vi "test_proceed.vi"() -> ()   [LabVIEW 2013]
uses:
  Classes/Flags/flag.lvclass
  global variables.vi
panel:
  in  "notifier name":string="test"
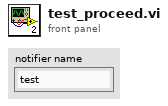
[diagram p1: front panel]
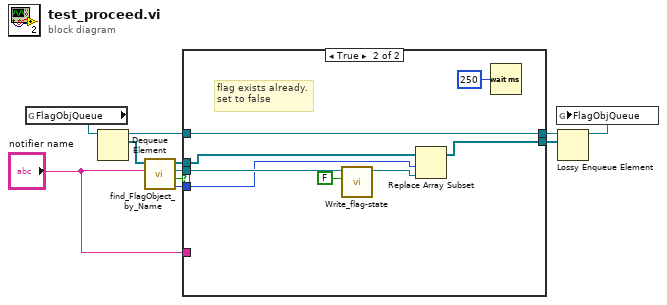
[diagram p0: block diagram]
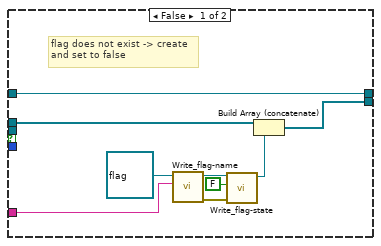
[diagram p2: hidden frame]
diagram:
  n1 = global read "global variables.vi" "FlagObjQueue"() -> (w11:refnum<queue>)
  n2 = Dequeue Element(queue=w11) -> (queue out=w9:refnum<queue>, element=w4:refnum<class "flag.lvclass">[])  [unwired: 2 in, 2 out]
  n3 = call "find_FlagObject_by_Name.vi"("Flag Name"="notifier name", "FlagObj Array"=w4) -> ("index of Object in Array"=w2:i32, "found?"=w10:bool, "found FlagObj out"=w7:refnum<class "flag.lvclass">, "FlagObj Array out"=w8:refnum<class "flag.lvclass">[])  [unwired: 6 in]
  n4 = case shown="True" w10 {
    tunnel: w9 -> [w13 w27]
    tunnel: w8 -> [w19 w24]
    tunnel: "notifier name" -> [w20 _]
    tunnel: w7 -> [_ w26]
    tunnel: [w13 w27] -> w6
    tunnel: [w12 w21] -> w5
    tunnel: w2 -> [_ w22]
    frame False {
      # "flag does not exist -> create\nand set to false"
      n5 = call-dynamic "Write_flag-name.vi"("flag name"=w20, "flag in"=refnum<class "flag.lvclass"> refnum ("flag.lvclass")) -> ("error out"=w16:errorcluster, "flag out"=w17:refnum<class "flag.lvclass">)  [unwired: 8 in]
      n6 = call-dynamic "Write_flag-state.vi"("error in (no error)"=w16, "flag state"=FALSE, "flag in"=w17) -> ("flag out"=w14:refnum<class "flag.lvclass">)  [unwired: 7 in, 1 out]
      n7 = Build Array (concatenate)(w19, w14) -> (w12:refnum<class "flag.lvclass">[])
    }
    frame True {
      # "flag exists already.\nset to false"
      n8 = call-dynamic "Write_flag-state.vi"("flag state"=FALSE, "flag in"=w26) -> ("flag out"=w23:refnum<class "flag.lvclass">)  [unwired: 8 in, 1 out]
      n9 = Replace Array Subset(array=w24, new element=w23, index=w22) -> (w21:refnum<class "flag.lvclass">[])
      n10 = Wait (ms)(milliseconds to wait=u32 250) -> ()  [unwired: 1 out]
    }
  }
  n11 = Lossy Enqueue Element(queue=w6, element=w5) -> (queue out=w3:refnum<queue>)  [unwired: 1 in, 3 out]
  n12 = global write "global variables.vi" "FlagObjQueue"(w3) -> ()
